vi "R1pHControl_Manual.vi"(7 "LabVIEW Web Service Request":refnum<class "Web Request.lvclass">, 9 "BasePump":bool, 11 "AcidPump":bool) -> (2 "ControlStatus":string, 3 "pH_Manual_Out":T1)   [LabVIEW 2016]
uses:
  <vilib>/wsapi/Web Request.lvclass
  Controls/pH_Manual Standard.ctl
panel:
  # "Use the Web Service Request input terminal to call the VIs on the Web Services palette. Do not remove it from the connector pane unless you don't need access to the palette."
  # "Each additional control wired to the connector pane will be available as an input in the URL. To include an indicator in terminal-mode output (the default setting), it must also be wired to the connector pane."
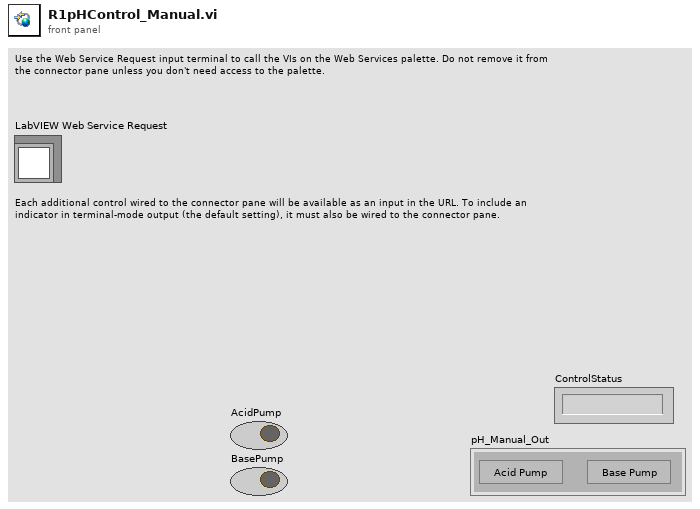
[diagram p1: front panel]
types:
  T1 = typedef "pH_Manual Standard.ctl" = cluster{"Acid Pump":bool, "Base Pump":bool}
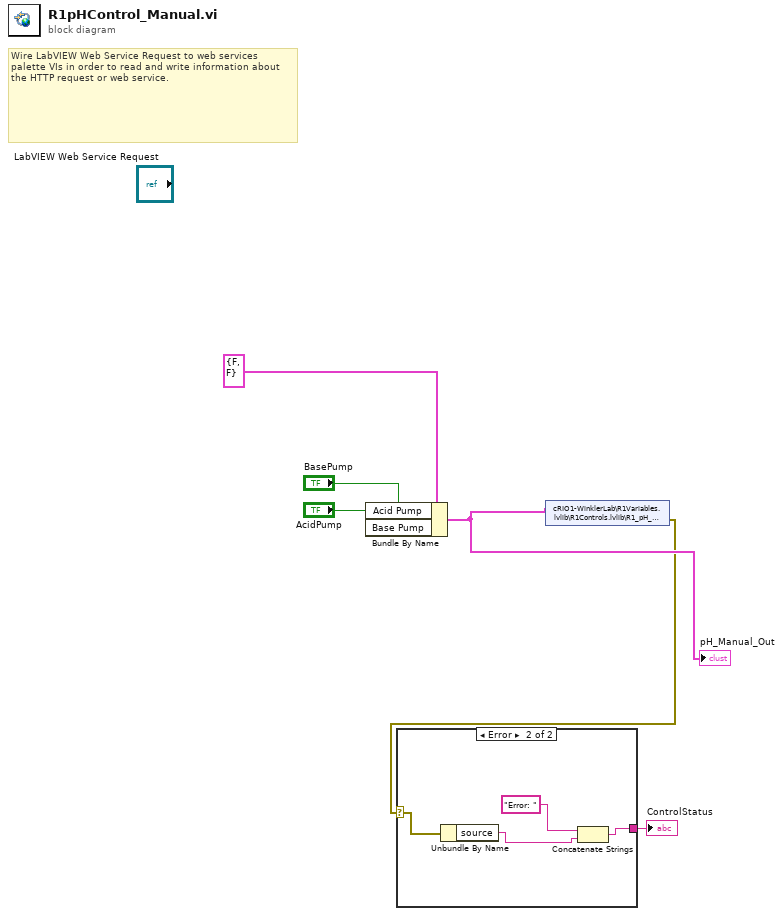
[diagram p0: block diagram]
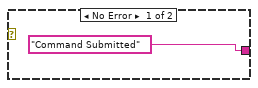
[diagram p2: hidden frame]
diagram:
  # "Wire LabVIEW Web Service Request to web services palette VIs in order to read and write information about the HTTP request or web service."
  n1 = Bundle By Name(cluster=T1 {"Acid Pump"=FALSE, "Base Pump"=FALSE} ("R1_pH_Manual"), "Acid Pump"="AcidPump", "Base Pump"="BasePump") -> (w5:T1)
  "pH_Manual_Out" <- w5
  n2 = shared-variable "cRIO1-WinklerLab\\R1Variables.lvlib\\R1Controls.lvlib\\R1_pH_Manual"(w5) -> (error out=w2:errorcluster)  [unwired: 1 in]
  n3 = case shown="Error" w2 {
    selector: w2 -> [_ w9]
    tunnel: ["Command Submitted" ("ControlStatus") w8] -> w1
    frame No Error {
    }
    frame Error {
      n4 = Unbundle By Name(w9) -> ("source"=w10:string)
      n5 = Concatenate Strings("Error: ", w10) -> (w8:string)
    }
  }
  "ControlStatus" <- w1
